vi "Download Submission.vi"(8 "error in (no error)":errorcluster, 11 "submission":i32) -> (0 "error out":errorcluster, 3 "Zip Path":path, 5 "Profile URL":string)   [LabVIEW 2024, in "Wordle Scorer.lvlib"]
uses:
  Wordle Scorer.lvlib
  Next Scoring Request.ctl
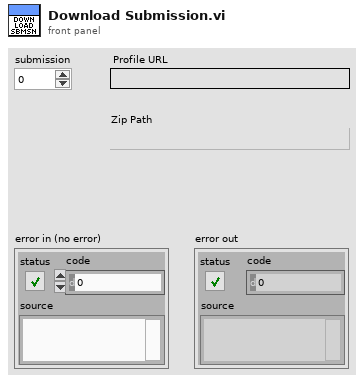
[diagram p1: front panel]
types:
  T1 = typedef "Wordle Scorer.lvlib/Next Scoring Request.ctl" = cluster{"scorer":string, "key":string, "challenges":i32[]}
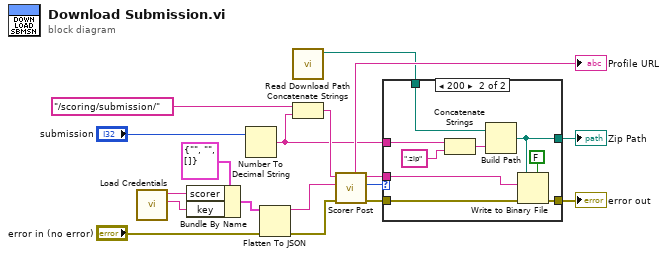
[diagram p0: block diagram]
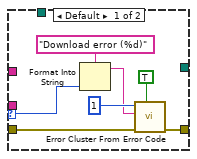
[diagram p2: hidden frame]
diagram:
  n1 = call "Load Credentials.vi"() -> ("Key"=w5:string, "ID"=w6:string)  [unwired: 9 in, 1 out]
  n2 = Bundle By Name(cluster=T1 {"scorer"="", "key"="", "challenges"=[]} ("Next Scoring Request"), "scorer"=w6, "key"=w5) -> (w4:T1)
  n3 = Number To Decimal String(number="submission") -> (decimal integer string=w10:string)  [unwired: 1 in]
  n4 = Flatten To JSON(anything=w4, error in (no error)="error in (no error)") -> (JSON string=w1:string, 11:w2:errorcluster)  [unwired: 1 in]
  n5 = call "Read Download Path.vi"() -> ("Download Path"=w14:path)  [unwired: 10 in, 1 out]
  n6 = Concatenate Strings("/scoring/submission/" ("format string"), w10) -> (w11:string)
  n7 = call "Scorer Post.vi"("error in (no error)"=w2, "buffer"=w1, "Path"=w11) -> ("error out"=w17:errorcluster, "Status"=w16:i32, "Content"=w15:string, "Profile URL"=→"Profile URL":string)  [unwired: 5 in]
  n8 = case shown="200" w16 {
    selector: w16 -> [w21 _]
    tunnel: w17 -> [w25 w30]
    tunnel: w15 -> [_ w29]
    tunnel: w14 -> [_ w31]
    tunnel: w10 -> [_ w34]
    tunnel: [w24 w27] -> w9
    tunnel: [_ w26] -> w8
    frame Default {
      n9 = Format Into String(format string="Download error (%d)", w21) -> (resulting string=w19:string)  [unwired: 2 in, 1 out]
      n10 = call <vilib>:"Error Cluster From Error Code.vi"("show call chain? (False)"=TRUE, "error in (no error)"=w25, "error message (\"\")"=w19, "error code (0)"=1) -> ("error out"=w24:errorcluster)  [unwired: 5 in]
    }
    frame 200 {
      n11 = Concatenate Strings(w34, ".zip" ("string")) -> (w32:string)
      n12 = Build Path(base path=w31, name or relative path=w32) -> (appended path=w26:path)
      n13 = Write to Binary File(file (use dialog)=w26, data=w29, error in=w30, 5:FALSE ("prepend array or string size? (T)")) -> (error out=w27:errorcluster)  [unwired: 2 in, 2 out]
    }
  }
  "error out" <- w9
  "Zip Path" <- w8
